vi "Word_Set_Font.vi"(0 "Range in":refnum<k7>, 2 "font":T1 {"font size" format="%.2f"; "strike through" items=["Unchanged", "Yes", "No"]; "underline" items=["Unchanged", "Yes", "No"]; "italic" items=["Unchanged", "Yes", "No"]; "bold" items=["Unchanged", "Yes", "No"]}, 3 "Error in":errorcluster) -> (6 "Range out":refnum<k7>, 9 "Error out":errorcluster)   [LabVIEW 2020, in "NI_ReportGenerationToolkit.lvlib"]
uses:
  <vilib>/addons/_office/NI_ReportGenerationToolkit.lvlib
  <vilib>/addons/_office/_exclsub.llb/font.ctl
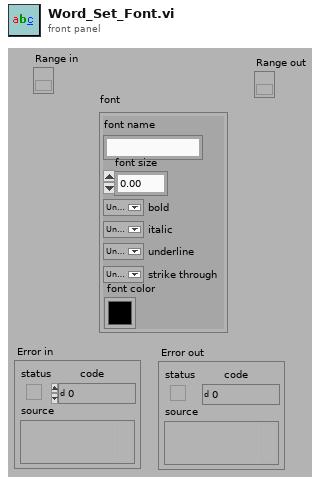
[diagram p1: front panel]
types:
  T1 = typedef "NI_ReportGenerationToolkit.lvlib/font.ctl" = cluster{"font name":string, "font size":dbl, "bold":u16, "italic":u16, "underline":u16, "strike through":u16, "font color":u32}
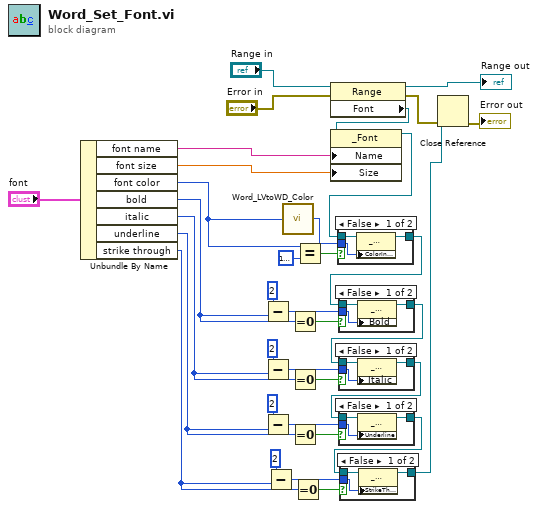
[diagram p0: block diagram]
diagram:
  n1 = Unbundle By Name("font") -> ("font name"=w29:string, "font size"=w28:dbl, "font color"=w1:u32, "bold"=w23:u16, "italic"=w13:u16, "underline"=w12:u16, "strike through"=w11:u16)
  n2 = Subtract(x=2, y=w23) -> (x-y=w24:i32)
  n3 = Subtract(x=2, y=w13) -> (x-y=w22:i32)
  n4 = Subtract(x=2, y=w12) -> (x-y=w17:i32)
  n5 = Subtract(x=2, y=w11) -> (x-y=w16:i32)
  n6 = call <vilib>:"Word_LVtoWD_Color.vi"("LabVIEW color"=w1) -> ("word color table index"=w3:i32)
  n7 = Equal To 0?(x=w23) -> (x = 0?=w27:bool)
  n8 = Equal To 0?(x=w13) -> (x = 0?=w20:bool)
  n9 = Equal To 0?(x=w12) -> (x = 0?=w19:bool)
  n10 = Equal To 0?(x=w11) -> (x = 0?=w14:bool)
  n11 = Equal?(x=w1, y=u32 16777216) -> (x = y?=w6:bool)
  n12 = property class="Range"(reference="Range in", error in="Error in") -> (reference out=→"Range out":refnum<k7>, error out=w31:errorcluster, "Font"=w35:refnum<k7>)
  n13 = property class="_Font"(reference=w35, "Name"=w29, "Size"=w28) -> (reference out=w5:refnum<k7>)  [unwired: 1 in, 1 out]
  n14 = case shown="False" w6 {
    tunnel: w5 -> [w38 w39]
    tunnel: w3 -> [w37 _]
    tunnel: [w36 w39] -> w4
    frame False {
      n15 = property class="_Font"(reference=w38, "ColorIndex"=w37) -> (reference out=w36:refnum<k7>)  [unwired: 1 in, 1 out]
    }
    frame True {
    }
  }
  n16 = case shown="False" w27 {
    tunnel: w4 -> [w42 w43]
    tunnel: w24 -> [w41 _]
    tunnel: [w40 w43] -> w10
    frame False {
      n17 = property class="_Font"(reference=w42, "Bold"=w41) -> (reference out=w40:refnum<k7>)  [unwired: 1 in, 1 out]
    }
    frame True {
    }
  }
  n18 = case shown="False" w20 {
    tunnel: w10 -> [w46 w47]
    tunnel: w22 -> [w45 _]
    tunnel: [w44 w47] -> w9
    frame False {
      n19 = property class="_Font"(reference=w46, "Italic"=w45) -> (reference out=w44:refnum<k7>)  [unwired: 1 in, 1 out]
    }
    frame True {
    }
  }
  n20 = case shown="False" w19 {
    tunnel: w9 -> [w50 w51]
    tunnel: w17 -> [w49 _]
    tunnel: [w48 w51] -> w8
    frame False {
      n21 = property class="_Font"(reference=w50, "Underline"=w49) -> (reference out=w48:refnum<k7>)  [unwired: 1 in, 1 out]
    }
    frame True {
    }
  }
  n22 = case shown="False" w14 {
    tunnel: w8 -> [w54 w55]
    tunnel: w16 -> [w53 _]
    tunnel: [w52 w55] -> w7
    frame False {
      n23 = property class="_Font"(reference=w54, "StrikeThrough"=w53) -> (reference out=w52:refnum<k7>)  [unwired: 1 in, 1 out]
    }
    frame True {
    }
  }
  n24 = Close Reference(reference=w7, error in (no error)=w31) -> (error out=→"Error out":errorcluster)
